vi "Write RawXML.vi"(8 "error in (no error)":errorcluster, 10 "RawXML":string, 11 "ParseSVG.lvclass":refnum<class "ParseSVG.lvclass">) -> (0 "error out":errorcluster, 3 "ParseSVG.lvclass 2":refnum<class "ParseSVG.lvclass">)   [LabVIEW 2019, in "ParseSVG.lvclass"]
uses:
  ParseSVG.lvclass
  ParseSVG.lvclass/ParseSVG.ctl
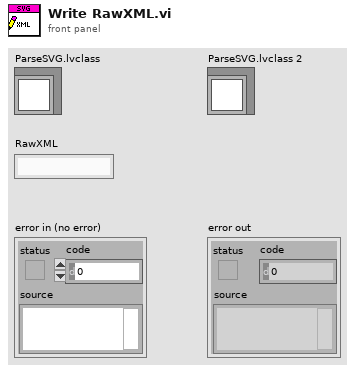
[diagram p1: front panel]
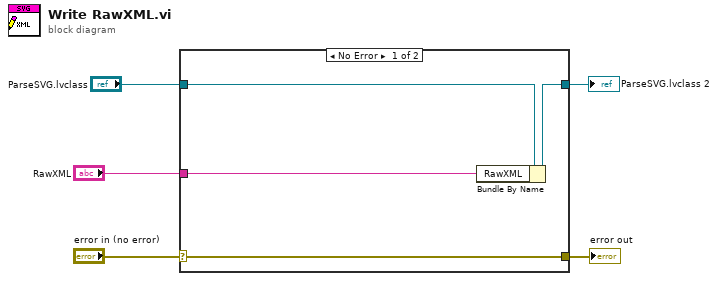
[diagram p0: block diagram]
diagram:
  n1 = case shown="No Error" "error in (no error)" {
    selector: "error in (no error)" -> [w9 w10]
    tunnel: [w9 w10] -> w4
    tunnel: [w6 w11] -> w1
    tunnel: "ParseSVG.lvclass" -> [w7 w11]
    tunnel: "RawXML" -> [w8 _]
    frame No Error {
      n2 = Bundle By Name(cluster=w7, "RawXML"=w8) -> (w6:refnum<class "ParseSVG.lvclass">)
    }
    frame Error {
    }
  }
  "error out" <- w4
  "ParseSVG.lvclass 2" <- w1
